vi "CLD 4 Event Structure Time Out Front Panel.vi"() -> ()   [LabVIEW 2025]
doc: "CLD 4 exercise"
panel:
  in  "Decrement":bool
  out "Error Out":errorcluster
  in  "Error In":errorcluster
  out "Time Has Elapsed":bool
  out "Count":string="0"
  in  "Increment":bool
  in  "Stop VI":bool
  in  "Timeout Target (s)":dbl=2.0
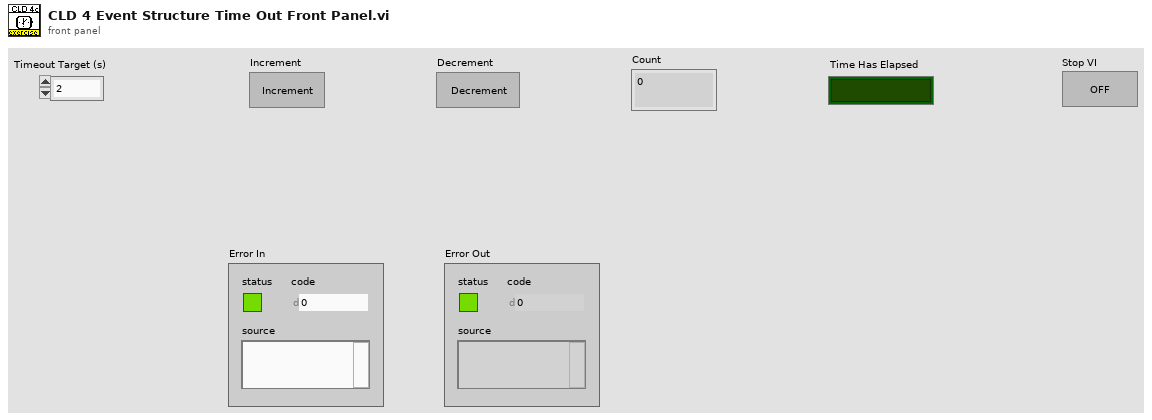
[diagram p1: front panel]
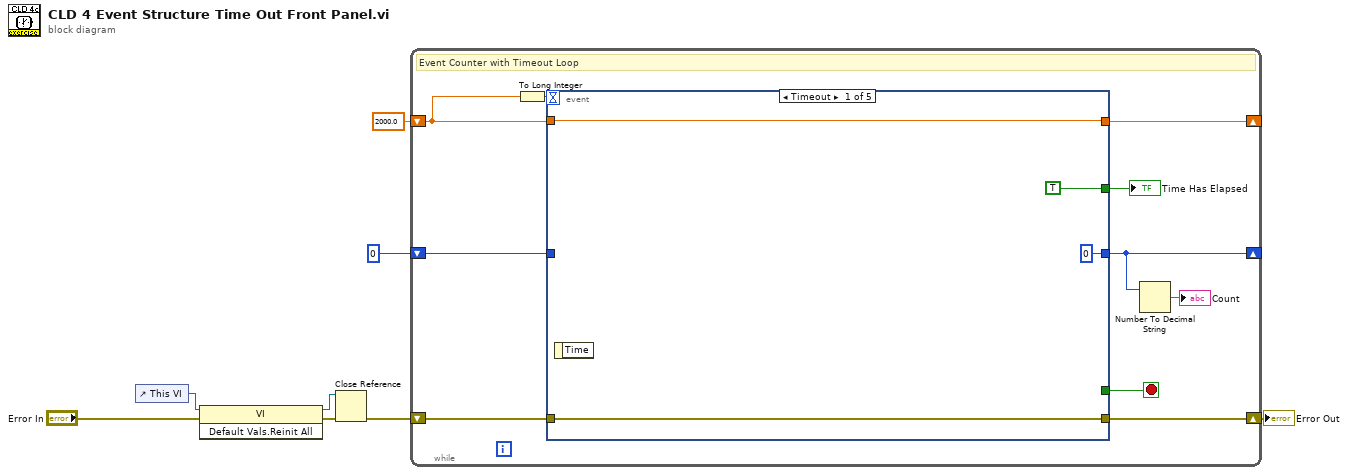
[diagram p0: block diagram]
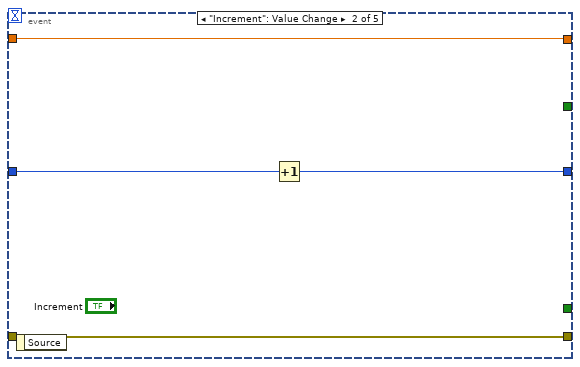
[diagram p2: hidden frame]
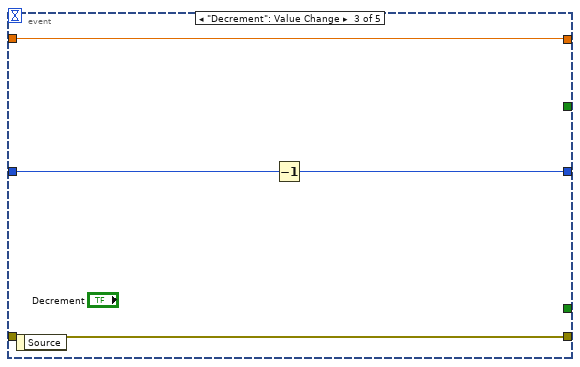
[diagram p3: hidden frame]
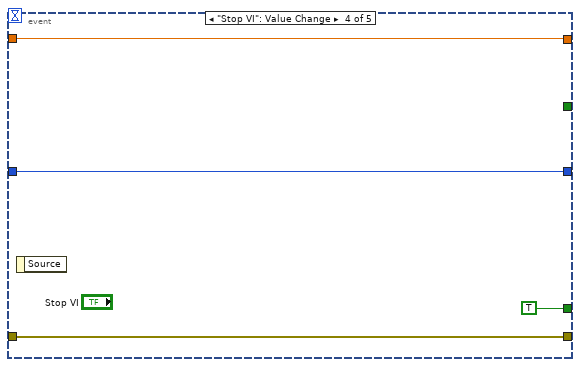
[diagram p4: hidden frame]
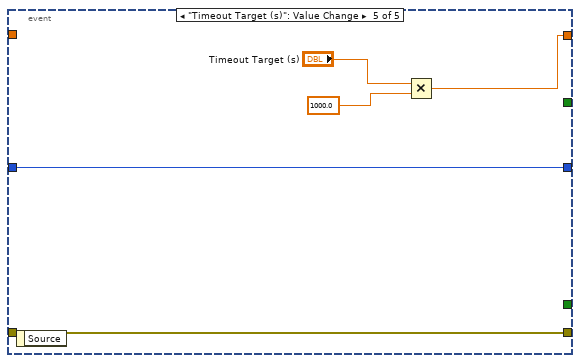
[diagram p5: hidden frame]
diagram:
  n1 = control-ref of="This VI"() -> (w3:refnum<vi>)
  n2 = invoke class="VI" method="Default Vals.Reinit All"(reference=w3, error in="Error In") -> (reference out=w1:refnum<vi>, error out=w4:errorcluster)  [unwired: 1 in, 1 out]
  n3 = Close Reference(reference=w1, error in (no error)=w4) -> (error out=w2:errorcluster)
  n4 = while {
    shift-right: [w17] -> w7
    shift-left: w2 -> [w18]
    shift-right: [w11] -> _
    shift-left: 2000.0 -> [w10]
    shift-right: [w14] -> _
    shift-left: u32 0 -> [w15]
    stop <- w12 stop-if-true
    # "Event Counter with Timeout Loop"
    n5 = To Long Integer(number=w10) -> (32bit integer=w16:i32)
    n6 = event shown="[0] Timeout" {
      selector: _ -> [_ _ _ _ _]
      dyn-events: _ -> [_ _ _ _ _]
      timeout: w16 -> [_ _ _ _ _]
      tunnel: w18 -> [w22 w24 w28 w33 w39]
      tunnel: [w22 w24 w28 w33 w39] -> w17
      tunnel: w15 -> [_ w26 w30 w34 w38]
      tunnel: [u32 0 w25 w29 w34 w38] -> w14
      tunnel: [_ _ _ TRUE _] -> w12
      tunnel: [w21 w23 w27 w31 w36] -> w11
      tunnel: w10 -> [w21 w23 w27 w31 _]
      tunnel: [TRUE _ _ _ _] -> w9
      event Timeout {
        n7 = event-data() -> ()  [unwired: 1 in, 1 out]
      }
      event "Increment": Value Change {
        n8 = event-data() -> ()  [unwired: 1 in, 1 out]
        n9 = Increment(x=w26) -> (x+1=w25:u32)
      }
      event "Decrement": Value Change {
        n10 = event-data() -> ()  [unwired: 1 in, 1 out]
        n11 = Decrement(x=w30) -> (x-1=w29:u32)
      }
      event "Stop VI": Value Change {
        n12 = event-data() -> ()  [unwired: 1 in, 1 out]
      }
      event "Timeout Target (s)": Value Change {
        n13 = event-data() -> ()  [unwired: 1 in, 1 out]
        n14 = Multiply(x="Timeout Target (s)", y=1000.0) -> (x*y=w36:dbl)
      }
    }
    "Time Has Elapsed" <- w9
    n15 = Number To Decimal String(number=w14) -> (decimal integer string=→"Count":string)  [unwired: 1 in]
  }
  "Error Out" <- w7
